vi "Visualisation.vi"() -> ()   [LabVIEW 2018]
uses:
  Lights Display.ctl
  States.ctl
  Color states.ctl
panel:
  out "Current state":T1=enum."Night"
  out "Color time 2":u32
  out "Color time 1":u32
  out "Traffic Lights 2":T2
  out "Traffic Lights 1":T2
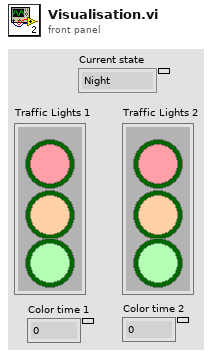
[diagram p1: front panel]
types:
  T1 = typedef "States.ctl" = enum16{"Normal", "Night", "Traffic jam 1", "Traffic jam 2"}
  T2 = typedef "Lights Display.ctl" = cluster{"Red":bool, "Amber":bool, "Green":bool}
  T3 = typedef "Color states.ctl" = enum16{"Green", "Red-Yellow", "Yellow", "Red", "Null"}
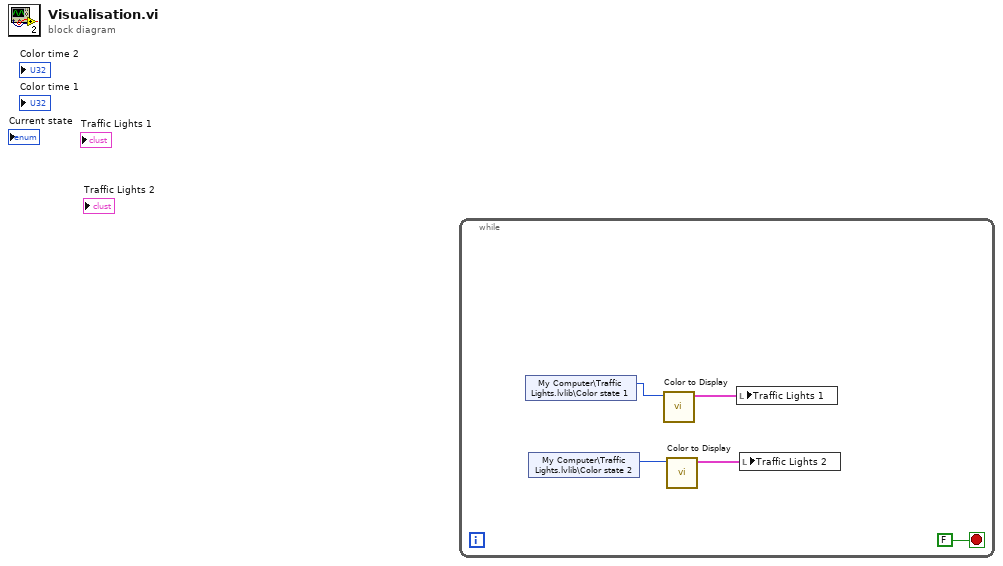
[diagram p0: block diagram]
diagram:
  n1 = while {
    stop <- FALSE stop-if-true
    n2 = shared-variable "My Computer\\Traffic Lights.lvlib\\Color state 1"() -> (w2:T3)  [unwired: 1 in, 1 out]
    n3 = shared-variable "My Computer\\Traffic Lights.lvlib\\Color state 2"() -> (w1:T3)  [unwired: 1 in, 1 out]
    n4 = call "Color to Display.vi"("Color state"=w2) -> ("Traffic Lights"=w5:T2)  [unwired: 10 in]
    n5 = call "Color to Display.vi"("Color state"=w1) -> ("Traffic Lights"=w3:T2)  [unwired: 10 in]
    n6 = local write "Traffic Lights 1"(w5) -> ()
    n7 = local write "Traffic Lights 2"(w3) -> ()
  }
